vi "Open Admin Tools.vi"(8 "error in (no error)":errorcluster, 11 "Data":variant) -> (0 "error out":errorcluster)   [LabVIEW 2018]
doc: "This subVI enqueues the named action in to the communications queue along with the input data."
uses:
  Private Controls/Module Action.ctl
  File IO.lvlib
  Private Controls/Module Data.ctl
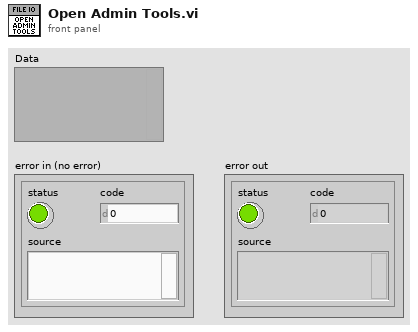
[diagram p1: front panel]
types:
  T1 = typedef "File IO.lvlib/Module Data.ctl" = cluster{"Data":variant, "Action":T2}
  T2 = typedef "File IO.lvlib/Module Action.ctl" = enum8{"Timeout", "Init", "Error", "Exit", "CreateOpen Data File", "Open Admin Tools", "Save Calibration Data", "Crash Log", "Set Testing State", "Set Recording State", "Set Test Information", "Set Sample Rate", "Set Username", "-----------Reporting-----------", "-------------TDMS -------------", "Check for Data", "Close Data File", "Add to System Log", "----------APU Setup File--------", "Save Stored APU Data", "Load APU Setup File", "Increment Run Count", "Write To Report", "Flush TDMS to File", "Create Report", "Set Report Filepath", "Change TDMS Group Name"}
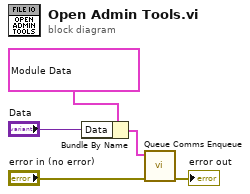
[diagram p0: block diagram]
diagram:
  n1 = Bundle By Name(cluster=T1 {"Data"=variant, "Action"=enum."Open Admin Tools"} ("element"), "Data"="Data") -> (w4:T1)
  n2 = call "Queue Comms Enqueue.vi"("error in (no error)"="error in (no error)", "element"=w4) -> ("error out"=→"error out":errorcluster)  [unwired: 9 in]
